vi "Write to File.vi"(8 "error in (no error)":errorcluster, 10 "INI Ref":T1, 11 "Image Assertion in":refnum<class "Image Assertion.lvclass">) -> (0 "error out":errorcluster, 2 "INI Ref out":T1, 3 "Image Assertion out":refnum<class "Image Assertion.lvclass">)   [LabVIEW 2020, in "MacroAssert.lvlib" / "Image Assertion.lvclass"]
uses:
  Image Assertion.lvclass
  Image Assertion.lvclass/Image Assertion.ctl
  MacroAssert.lvlib
  <vilib>/Utility/config.llb/NI_LVConfig.lvlib
  <vilib>/Utility/config.llb/Write Key (I32).vi
  <vilib>/Utility/config.llb/Write Key (String).vi
  Control Assertion/Control Assertion.lvclass
  <vilib>/Utility/config.llb/Config Data RefNum.ctl
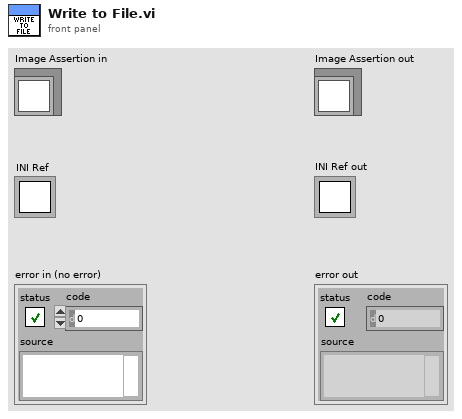
[diagram p1: front panel]
types:
  T1 = typedef "NI_LVConfig.lvlib/Config Data RefNum.ctl" = refnum<k1>
  T2 = typedef "imagedata.ctl" = cluster{"image type":i32, "image depth":i32, "image":u8[], "mask":u8[], "colors":u32[], "Rectangle":cluster{"left":i16, "top":i16, "right":i16, "bottom":i16}}
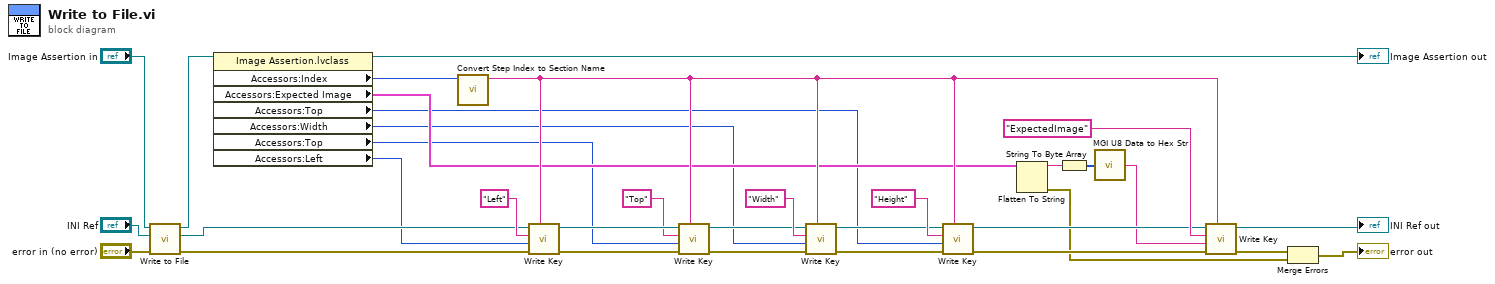
[diagram p0: block diagram]
diagram:
  n1 = call-parent "Write to File.vi"("error in (no error)"="error in (no error)", "INI Ref"="INI Ref", "Control Assertion in"="Image Assertion in") -> ("error out"=w26:errorcluster, "INI Ref out"=w23:T1, "Control Assertion out"=w25:refnum<class "Image Assertion.lvclass">)  [unwired: 6 in]
  n2 = property class="Image Assertion.lvclass"(reference=w25) -> (reference out=→"Image Assertion out":refnum<class "Image Assertion.lvclass">, "Accessors:Index"=w27:i32, "Accessors:Expected Image"=w7:T2, "Accessors:Top"=w3:i16, "Accessors:Width"=w4:i16, "Accessors:Top"=w5:i16, "Accessors:Left"=w6:i16)  [unwired: 1 in, 1 out]
  n3 = call "Convert Step Index to Section Name.vi"("Step Index"=w27) -> ("Section Name"=w11:string)  [unwired: 10 in]
  n4 = call-poly <vilib>:"Write Key.vi"("section"=w11, "error in (no error)"=w26, "value"=w6, "key"="Left", "refnum"=w23) -> ("error out"=w29:errorcluster, "refnum out"=w31:T1)  [unwired: 4 in, 1 out]
  n5 = call-poly <vilib>:"Write Key.vi"("section"=w11, "error in (no error)"=w29, "value"=w5, "key"="Top", "refnum"=w31) -> ("error out"=w17:errorcluster, "refnum out"=w18:T1)  [unwired: 4 in, 1 out]
  n6 = call-poly <vilib>:"Write Key.vi"("section"=w11, "error in (no error)"=w17, "value"=w4, "key"="Width", "refnum"=w18) -> ("error out"=w21:errorcluster, "refnum out"=w19:T1)  [unwired: 4 in, 1 out]
  n7 = call-poly <vilib>:"Write Key.vi"("section"=w11, "error in (no error)"=w21, "value"=w3, "key"="Height", "refnum"=w19) -> ("error out"=w14:errorcluster, "refnum out"=w15:T1)  [unwired: 4 in, 1 out]
  n8 = Flatten To String(anything=w7) -> (data string=w9:string, error out=w1:errorcluster)  [unwired: 3 in, 1 out]
  n9 = String To Byte Array(string=w9) -> (unsigned byte array=w8:u8[])
  n10 = call <userlib>:"MGI U8 Data to Hex Str.vi"("u8 Data[]"=w8) -> ("HEX String (0-9,A-F)"=w2:string)
  n11 = call-poly <vilib>:"Write Key.vi"("section"=w11, "error in (no error)"=w14, "value"=w2, "key"="ExpectedImage", "refnum"=w15) -> ("error out"=w12:errorcluster, "refnum out"=→"INI Ref out":T1)  [unwired: 4 in, 1 out]
  n12 = Merge Errors(w12, w1) -> (→"error out":errorcluster)
